vi "array_problem_6.vi"() -> ()   [LabVIEW 2020]
panel:
  out "product":dbl
  out "sum":dbl
  in  "Array":dbl[](array[numeric])
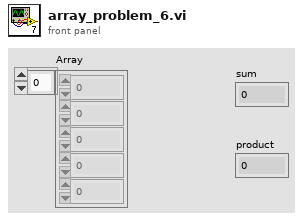
[diagram p1: front panel]
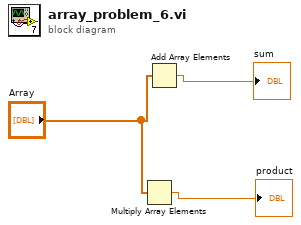
[diagram p0: block diagram]
diagram:
  n1 = Multiply Array Elements(1:"Array") -> (0:→"product":dbl)
  n2 = Add Array Elements(numeric array="Array") -> (sum=→"sum":dbl)
